vi "SetInstrumentHandle.vi"(8 "error in (no error)":errorcluster, 10 "Instrument Handle":u32, 11 "AnalogDiscoveryFunction in":refnum<class "AnalogDiscoveryFunction.lvclass">) -> (0 "error out":errorcluster, 3 "AnalogDiscoveryFunction out":refnum<class "AnalogDiscoveryFunction.lvclass">)   [LabVIEW 2020, in "AnalogDiscoveryFunction.lvclass"]
uses:
  AnalogDiscoveryFunction.lvclass
  AnalogDiscoveryFunction.lvclass/AnalogDiscoveryFunction.ctl
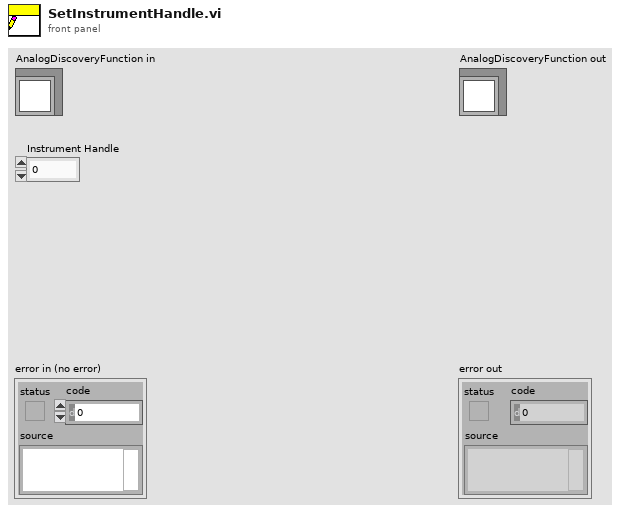
[diagram p1: front panel]
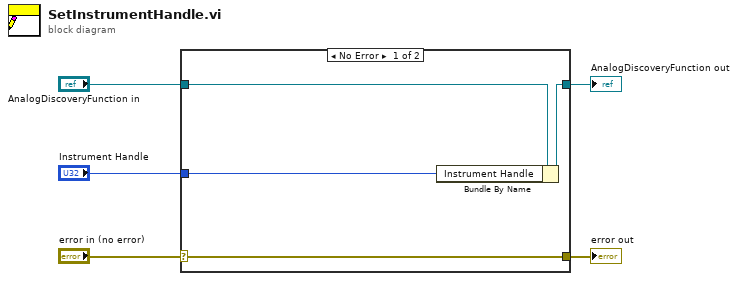
[diagram p0: block diagram]
diagram:
  n1 = case shown="No Error" "error in (no error)" {
    selector: "error in (no error)" -> [w9 w10]
    tunnel: [w9 w10] -> w4
    tunnel: [w7 w11] -> w2
    tunnel: "AnalogDiscoveryFunction in" -> [w8 w11]
    tunnel: "Instrument Handle" -> [w6 _]
    frame No Error {
      n2 = Bundle By Name(cluster=w8, "Instrument Handle"=w6) -> (w7:refnum<class "AnalogDiscoveryFunction.lvclass">)
    }
    frame Error {
    }
  }
  "error out" <- w4
  "AnalogDiscoveryFunction out" <- w2
